vi "define.vi"(8 "error in (no error)":errorcluster, 11 "TrajectoryDL090201FrameScan in":refnum<class "TrajectoryDL090201FrameScan.lvclass">) -> (0 "error out":errorcluster, 3 "TrajectoryDL090201FrameScan out":refnum<class "TrajectoryDL090201FrameScan.lvclass">)   [LabVIEW 2010, in "TrajectoryDL090201FrameScan.lvclass"]
doc: "modal dialog on which the user can set the trajectory parameters"
uses:
  TrajectoryDL090201FrameScan.lvclass
panel:
  in  "no. of offset pixels (Pockels cell closed)":i32
  in  "cancelButton":bool
  in  "okButton":bool
  in  "no. of pixels with Pockels cell closed":i32
  in  "no. of pixels with Pockels cell open":i32
  # "Define trajectory details"
  # "pixels per package"
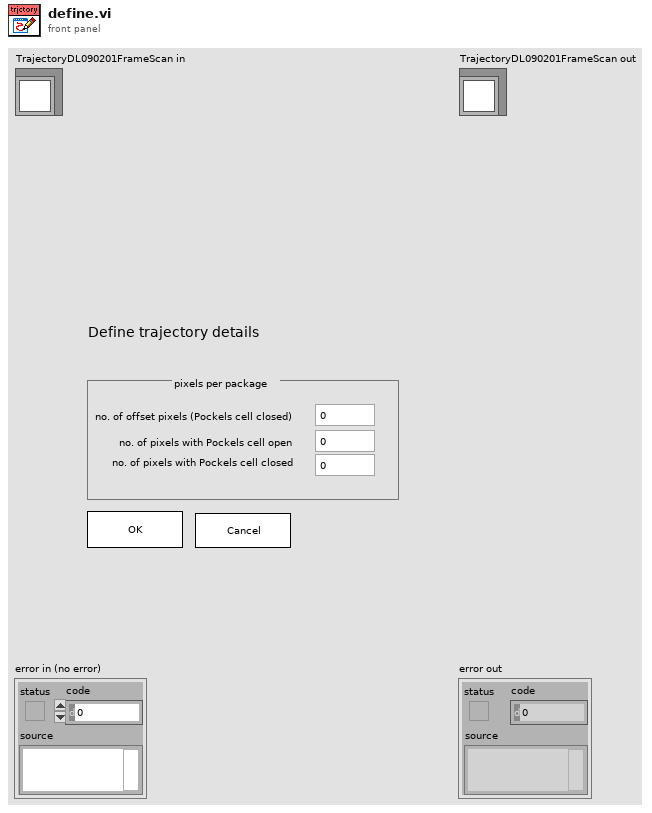
[diagram p1: front panel]
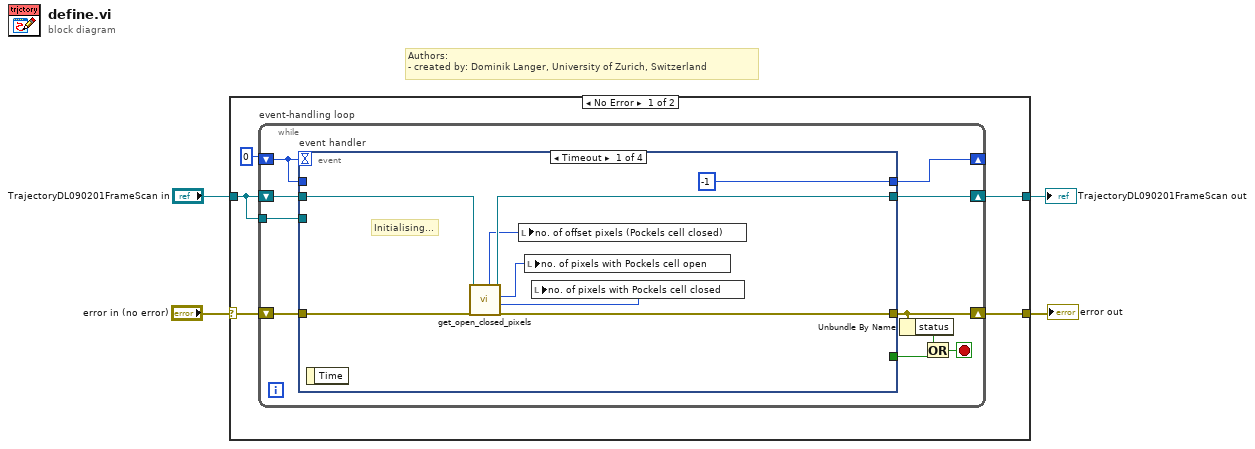
[diagram p0: block diagram]
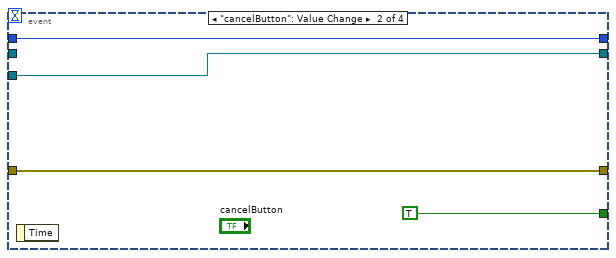
[diagram p2: hidden frame]
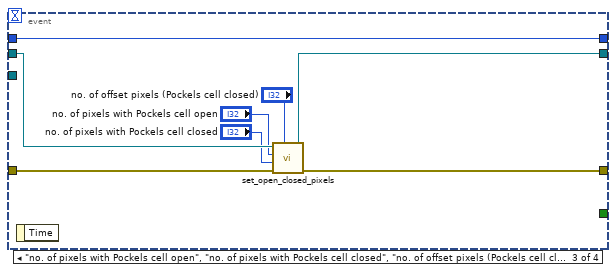
[diagram p3: hidden frame]
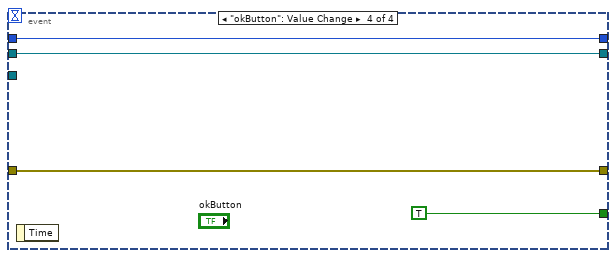
[diagram p4: hidden frame]
diagram:
  # "Authors: \n- created by: Dominik Langer, University of Zurich, Switzerland"
  n1 = case shown="No Error" "error in (no error)" {
    selector: "error in (no error)" -> [w9 w45]
    tunnel: "TrajectoryDL090201FrameScan in" -> [w6 w44]
    tunnel: [w8 w45] -> w2
    tunnel: [w7 w44] -> w1
    frame No Error {
      n2 = while "event-handling loop" {
        shift-right: [w17] -> w7
        shift-left: w6 -> [w18]
        shift-right: [w16] -> w8
        shift-left: w9 -> [w19]
        tunnel: w6 -> [w12]
        shift-right: [w10] -> _
        shift-left: 0 -> [w11]
        stop <- w15 stop-if-true
        n3 = event "event handler" shown="[0] Timeout" {
          selector: _ -> [_ _ _ _]
          dyn-events: _ -> [_ _ _ _]
          timeout: w11 -> [_ _ _ _]
          tunnel: w19 -> [w25 w31 w38 w43]
          tunnel: w18 -> [w23 _ w37 w42]
          tunnel: [w24 w31 w34 w43] -> w16
          tunnel: [w22 w29 w33 w42] -> w17
          tunnel: [_ TRUE _ TRUE] -> w14
          tunnel: w12 -> [_ w29 _ _]
          tunnel: w11 -> [_ w28 w39 w40]
          tunnel: [-1 w28 w39 w40] -> w10
          event Timeout {
            # "Initialising..."
            n4 = event-data() -> ()  [unwired: 1 in, 1 out]
            n5 = call-dynamic "get_open_closed_pixels.vi"("error in (no error)"=w25, "TrajectoryDL090201FrameScan in"=w23) -> ("error out"=w24:errorcluster, "number of closed pixels"=w21:i32, "number of open pixels"=w26:i32, "TrajectoryDL090201FrameScan out"=w22:refnum<class "TrajectoryDL090201FrameScan.lvclass">, "number of offset pixels"=w20:i32)  [unwired: 5 in]
            n6 = local write "no. of offset pixels (Pockels cell closed)"(w20) -> ()
            n7 = local write "no. of pixels with Pockels cell open"(w26) -> ()
            n8 = local write "no. of pixels with Pockels cell closed"(w21) -> ()
          }
          event "cancelButton": Value Change {
            n9 = event-data() -> ()  [unwired: 1 in, 1 out]
          }
          event "no. of pixels with Pockels cell open", "no. of pixels with Pockels cell closed", "no. of offset pixels (Pockels cell closed)": Value Change {
            n10 = event-data() -> ()  [unwired: 1 in, 1 out]
            n11 = call-dynamic "set_open_closed_pixels.vi"("number of offset pixels"="no. of offset pixels (Pockels cell closed)", "error in (no error)"=w38, "number of closed pixels"="no. of pixels with Pockels cell closed", "number of open pixels"="no. of pixels with Pockels cell open", "TrajectoryDL090201FrameScan in"=w37) -> ("error out"=w34:errorcluster, "TrajectoryDL090201FrameScan out"=w33:refnum<class "TrajectoryDL090201FrameScan.lvclass">)  [unwired: 5 in]
          }
          event "okButton": Value Change {
            n12 = event-data() -> ()  [unwired: 1 in, 1 out]
          }
        }
        n13 = Unbundle By Name(w16) -> ("status"=w13:bool)
        n14 = Or(x=w13, y=w14) -> (x .or. y?=w15:bool)
      }
    }
    frame Error {
    }
  }
  "error out" <- w2
  "TrajectoryDL090201FrameScan out" <- w1
